vi "AutofocusOptions_old.vi"() -> ()   [LabVIEW 2019]
uses:
  <vilib>/Utility/file.llb/Read Delimited Spreadsheet (DBL).vi
panel:
  in  "DistSensorInTextFileMode":bool
  out "XYZ_NiterOrDistSenErr":string
  in  "AbortAutoFocus":bool
  in  "Tolerance":dbl=0.005 format="%#_13g"
  out "TimeTaken":dbl
  out "Z":string
  in  "SafeMaxZ":dbl=75.0 format="%#_13g"
  out "N_iterations":dbl[](array[numeric])
  in  "InitialStepSize":dbl=0.1
  out "HighVSPosition":picture
  in  "Z OutputFile":path=path "C:/Users/TTUHEP/Documents/LabVIEW/GantryPrograms/LogFiles/temp.txt"
  in  "PlotOutputFile":string="C:\\Users\\TTUHEP\\Documents\\LabVIEW\\GantryPrograms\\LogFiles\\plot.png"
  in  "Zoffset_textFile":dbl
  out "Image":T1(plugin-control)
  in  "InitialPositions":path=path "C:/Users/TTUHEP/Documents/LabVIEW/GantryPrograms/Configs/A1_BP_HeightMeasure.txt"
  out "error out":errorcluster
  out "BestZvalue":dbl
  in  "error in (no error)":errorcluster
  in  "Z":dbl=68.683
  in  "Y":dbl=1011.604463
  in  "X":dbl=288.7508563
  in  "ControlType":T2(ring)=enum."SinglePoint" caption="Operation Mode"
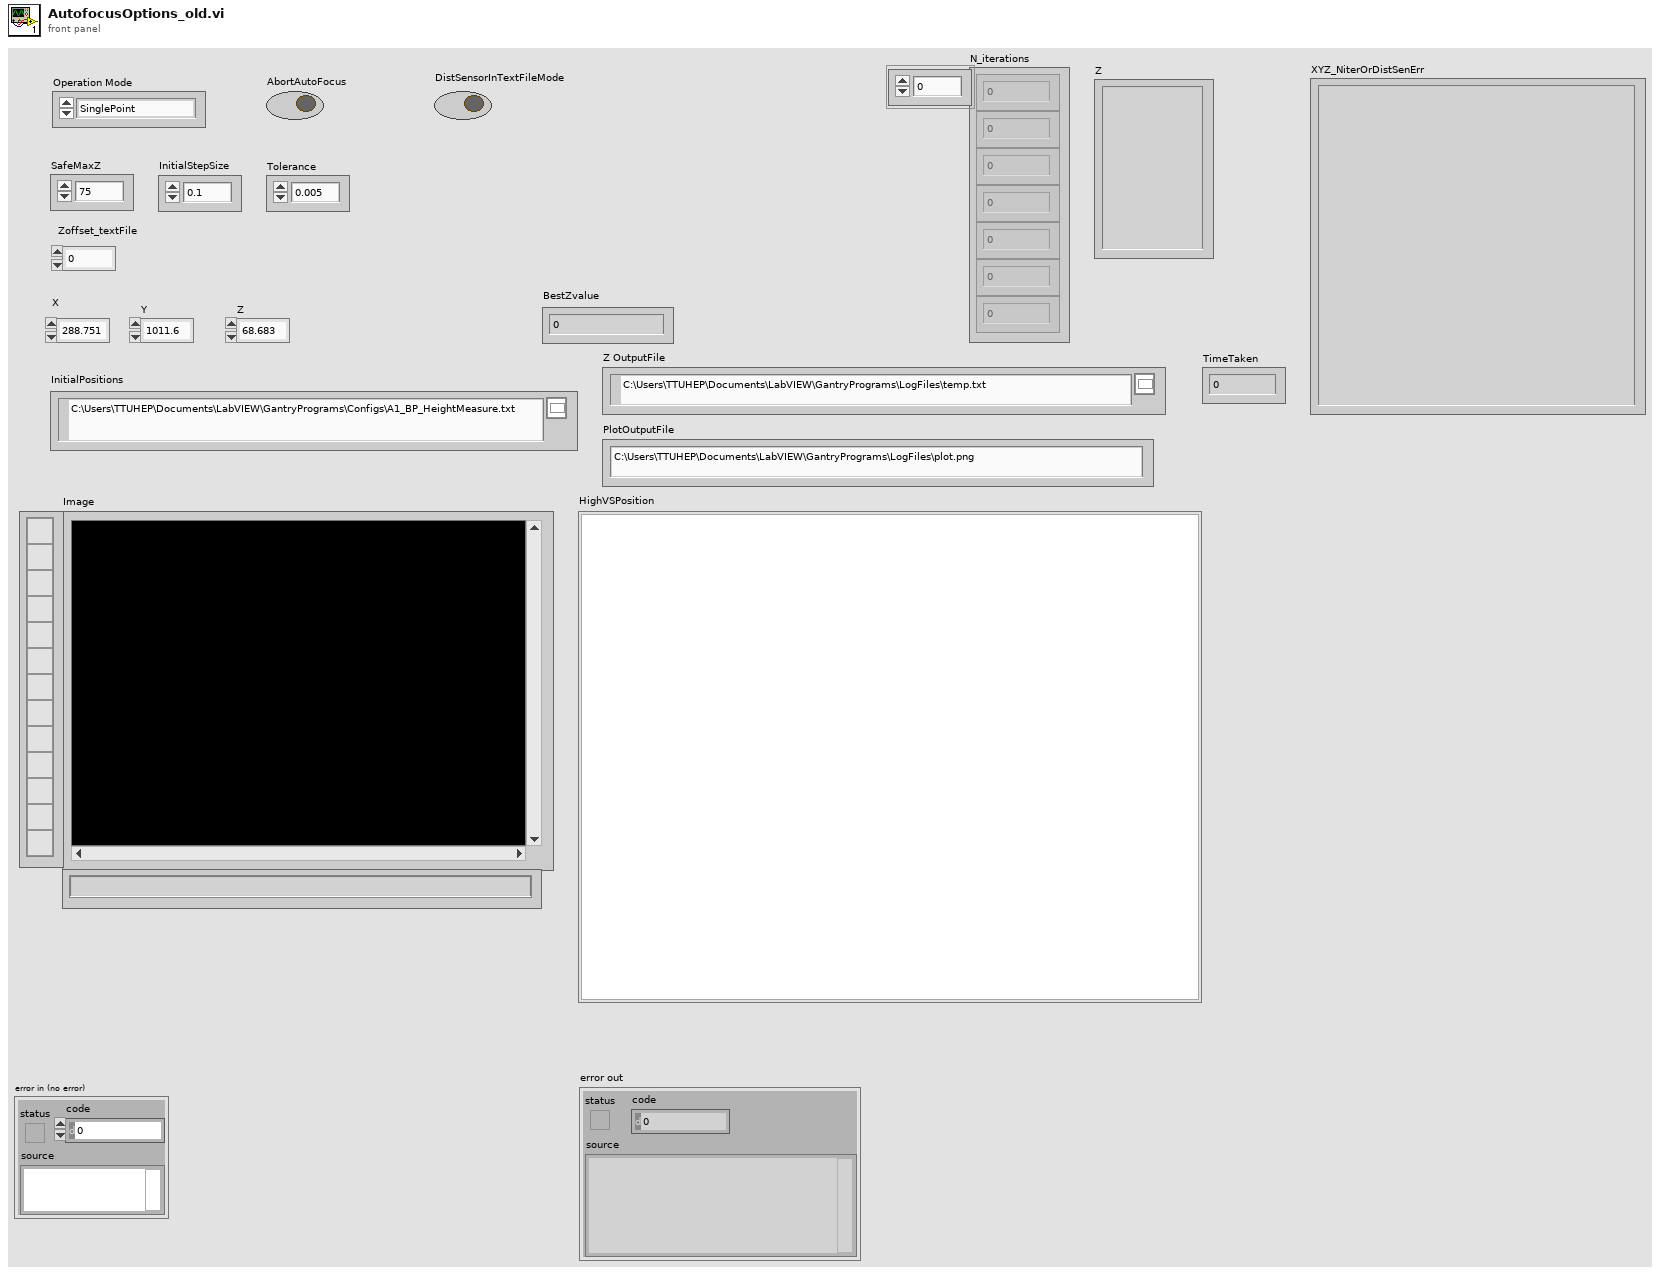
[diagram p1: front panel]
types:
  T1 = typedef "IMAQ Image.ctl" = refnum<image>
  T2 = enum16{"CurrentPosition", "SinglePoint", "TextFile"}
  T3 = enum16{"open", "replace", "create", "open or create", "replace or create", "replace or create with confirmation"}
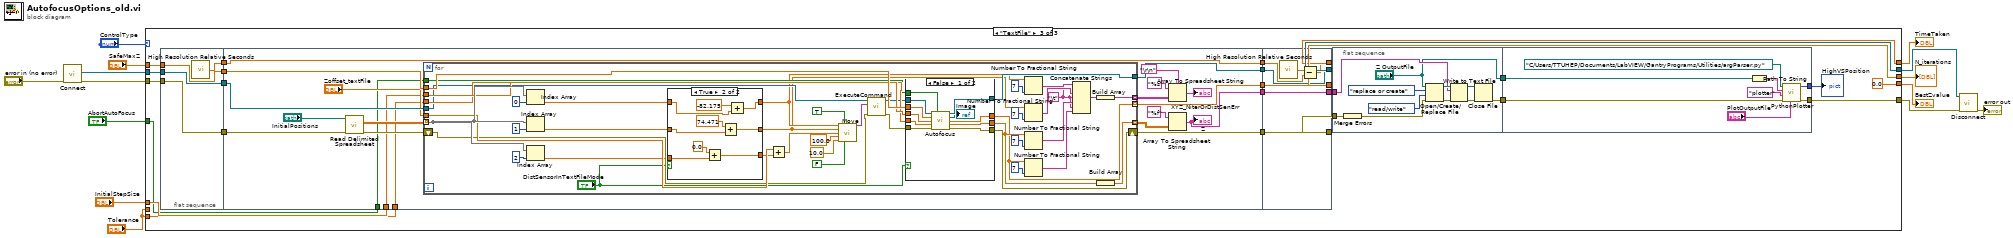
[diagram p0: block diagram]
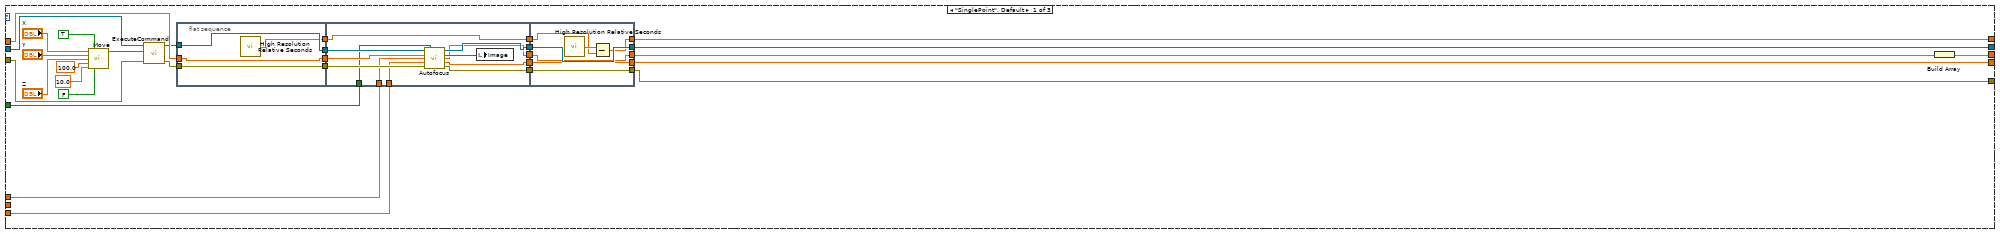
[diagram p2: hidden frame]
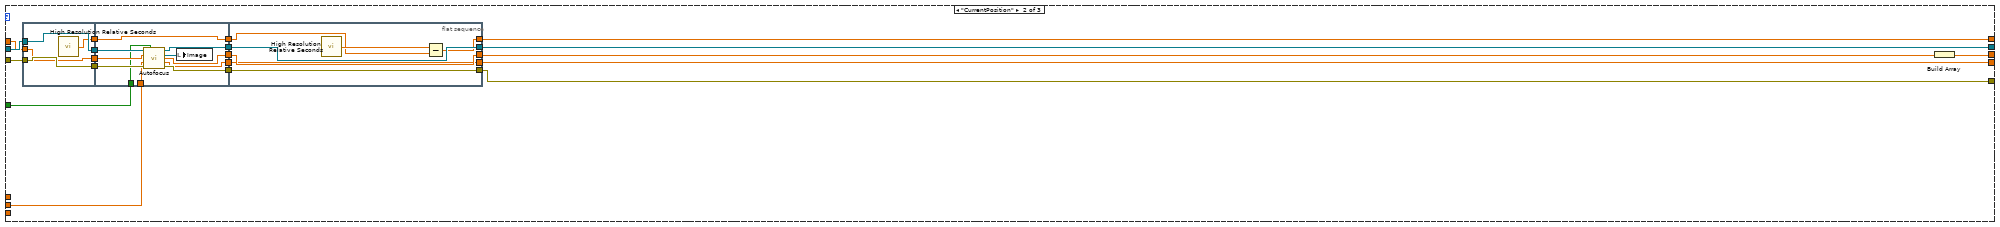
[diagram p3: hidden frame]
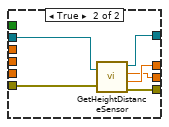
[diagram p4: hidden frame]
diagram:
  n1 = call "Connect.vi"("error in (no error)"="error in (no error)") -> ("error out"=w11:errorcluster, "controller"=w13:refnum<k24>)  [unwired: 9 in]
  n2 = case shown="\"TextFile\"" "ControlType" {
    tunnel: w11 -> [w19 w86 w130]
    tunnel: [w45 w82 w126] -> w10
    tunnel: w13 -> [w29 w87 w134]
    tunnel: [w44 w83 w133] -> w8
    tunnel: [w42 w84 w131] -> w7
    tunnel: "SafeMaxZ" -> [w41 w85 w129]
    tunnel: [w40 w81 0.0 ("BestZvalue")] -> w5
    tunnel: [w30 w71 w114] -> w4
    tunnel: "Tolerance" -> [_ w70 _]
    tunnel: "InitialStepSize" -> [w17 _ w113]
    tunnel: "Tolerance" -> [w16 _ w112]
    tunnel: "AbortAutoFocus" -> [w15 w69 w111]
    frame "SinglePoint", Default {
      n3 = call "Move.vi"("X"="X", "Absolute"=TRUE, "Y"="Y", "Z"="Z", "SpeedXY (mm/s)"=100.0, "SpeedZ (mm/s)"=10.0, "Move Z first"=FALSE) -> ("Position Gcode"=w20:string)  [unwired: 8 in]
      n4 = call "ExecuteCommand.vi"("error in (no error)"=w19, "Command Code"=w20, "controller in"=w29) -> ("error out"=w18:errorcluster, "controller out"=w28:refnum<k24>)  [unwired: 6 in, 1 out]
      n5 = flat-sequence {
        tunnel: w41 -> [w48]
        tunnel: w28 -> [w49]
        tunnel: [w46] -> w39
        tunnel: [w49] -> w38
        tunnel: [w48] -> w37
        tunnel: [w47] -> w31
        tunnel: w18 -> [w46]
        tunnel: w39 -> [w61]
        tunnel: w38 -> [w54]
        tunnel: w37 -> [w51]
        tunnel: [w60] -> w36
        tunnel: [w59] -> w35
        tunnel: [w57] -> w34
        tunnel: [w56] -> w33
        tunnel: [w55] -> w32
        tunnel: w31 -> [w55]
        tunnel: w17 -> [w53]
        tunnel: w16 -> [w52]
        tunnel: w15 -> [w50]
        tunnel: [w65] -> w40
        tunnel: [w66] -> w43
        tunnel: [w67] -> w44
        tunnel: [w68] -> w45
        tunnel: w36 -> [w68]
        tunnel: w35 -> [w67]
        tunnel: w34 -> [w66]
        tunnel: w33 -> [w65]
        tunnel: w32 -> [w63]
        tunnel: [w62] -> w30
        frame #0 {
          n6 = call <vilib>:"High Resolution Relative Seconds.vi"() -> ("relative seconds"=w47:dbl)
        }
        frame #1 {
          n7 = call "Autofocus.vi"("controller in"=w54, "AbortAutoFocus"=w50, "SafeMaxZ"=w51, "InitialStepSize"=w53, "Tolerance"=w52, "error in (no error)"=w61) -> ("controller out"=w59:refnum<k24>, "Image"=w58:T1, "N_iterations"=w57:dbl, "BestZvalue"=w56:dbl, "error out"=w60:errorcluster)  [unwired: 5 in]
          n8 = local write "Image"(w58) -> ()
        }
        frame #2 {
          n9 = call <vilib>:"High Resolution Relative Seconds.vi"() -> ("relative seconds"=w64:dbl)
          n10 = Subtract(x=w64, y=w63) -> (x-y=w62:dbl)
        }
      }
      n11 = Build Array(w43) -> (w42:dbl[])
    }
    frame "CurrentPosition" {
      n12 = flat-sequence {
        tunnel: w85 -> [w90]
        tunnel: w86 -> [w91]
        tunnel: w87 -> [w92]
        tunnel: [w92] -> w80
        tunnel: [w91] -> w79
        tunnel: [w90] -> w78
        tunnel: [w89] -> w73
        tunnel: w80 -> [w97]
        tunnel: w79 -> [w96]
        tunnel: w78 -> [w95]
        tunnel: [w102] -> w77
        tunnel: [w101] -> w76
        tunnel: [w100] -> w75
        tunnel: [w99] -> w74
        tunnel: w73 -> [w98]
        tunnel: [w98] -> w72
        tunnel: w70 -> [w94]
        tunnel: w69 -> [w93]
        tunnel: [w107] -> w81
        tunnel: [w108] -> w82
        tunnel: [w109] -> w83
        tunnel: [w110] -> w88
        tunnel: w77 -> [w110]
        tunnel: w76 -> [w109]
        tunnel: w75 -> [w108]
        tunnel: w74 -> [w107]
        tunnel: w72 -> [w105]
        tunnel: [w104] -> w71
        frame #0 {
          n13 = call <vilib>:"High Resolution Relative Seconds.vi"() -> ("relative seconds"=w89:dbl)
        }
        frame #1 {
          n14 = call "Autofocus.vi"("controller in"=w97, "AbortAutoFocus"=w93, "SafeMaxZ"=w95, "Tolerance"=w94, "error in (no error)"=w96) -> ("controller out"=w101:refnum<k24>, "Image"=w103:T1, "N_iterations"=w102:dbl, "BestZvalue"=w99:dbl, "error out"=w100:errorcluster)  [unwired: 6 in]
          n15 = local write "Image"(w103) -> ()
        }
        frame #2 {
          n16 = call <vilib>:"High Resolution Relative Seconds.vi"() -> ("relative seconds"=w106:dbl)
          n17 = Subtract(x=w106, y=w105) -> (x-y=w104:dbl)
        }
      }
      n18 = Build Array(w88) -> (w84:dbl[])
    }
    frame "TextFile" {
      n19 = flat-sequence {
        tunnel: w129 -> [w137]
        tunnel: w130 -> [w138]
        tunnel: w134 -> [w139]
        tunnel: [w139] -> w123
        tunnel: [w138] -> w122
        tunnel: [w137] -> w121
        tunnel: [w136] -> w116
        tunnel: w123 -> [w158]
        tunnel: w122 -> [w154]
        tunnel: w121 -> [w152]
        tunnel: [w140] -> w120
        tunnel: [w157] -> w119
        tunnel: [w141] -> w118
        tunnel: [w155] -> w117
        tunnel: w116 -> [w149]
        tunnel: [w149] -> w115
        tunnel: w113 -> [w148]
        tunnel: w112 -> [w147]
        tunnel: w111 -> [w146]
        tunnel: [w235] -> w131
        tunnel: [w236] -> w132
        tunnel: [w237] -> w133
        tunnel: [w238] -> w135
        tunnel: w120 -> [w238]
        tunnel: w119 -> [w237]
        tunnel: w118 -> [w236]
        tunnel: w117 -> [w235]
        tunnel: w115 -> [w233]
        tunnel: [w232] -> w114
        frame #0 {
          n20 = call <vilib>:"High Resolution Relative Seconds.vi"() -> ("relative seconds"=w136:dbl)
        }
        frame #1 {
          n21 = call-poly <vilib>:"Read Delimited Spreadsheet.vi"("file path (dialog if empty)"="InitialPositions", "error in (no error)"=w154) -> ("all rows"=w160:dbl[][], "error out"=w153:errorcluster)  [unwired: 8 in, 4 out]
          n22 = for {
            tunnel: w160 -> [w199] mode=indexing
            tunnel: [w198] -> w150 mode=indexing
            tunnel: w158 -> [w184]
            tunnel: [w197] -> w157
            tunnel: [w163] -> w155 mode=indexing
            tunnel: w152 -> [w187]
            tunnel: "Zoffset_textFile" -> [w196]
            tunnel: w148 -> [w186]
            tunnel: w147 -> [w185]
            tunnel: w146 -> [w182]
            tunnel: [w173] -> w145 mode=indexing
            shift-right: [w172] -> w140
            shift-left: w153 -> [w189]
            w164 = "\t"
            n23 = Index Array(array=w199, index=0) -> (element=w170:dbl)
            n24 = Index Array(array=w199, index=1) -> (element=w168:dbl)
            n25 = Index Array(array=w199, index=2) -> (element=w167:dbl)
            n26 = case shown="True" "DistSensorInTextFileMode" {
              tunnel: [w222 w230] -> w171
              tunnel: w170 -> [w222 w229]
              tunnel: [w221 w228] -> w169
              tunnel: w168 -> [w221 w226]
              tunnel: w167 -> [w220 w225]
              tunnel: [w220 w223] -> w166
              frame False {
              }
              frame True {
                n27 = Add(x=0.0, y=w225) -> (x+y=w223:dbl)
                n28 = Add(x=74.471, y=w226) -> (x+y=w228:dbl)
                n29 = Add(x=-82.175, y=w229) -> (x+y=w230:dbl)
              }
            }
            n30 = Add(x=w196, y=w166) -> (x+y=w195:dbl)
            n31 = call "Move.vi"("X"=w171, "Absolute"=TRUE, "Y"=w169, "Z"=w195, "SpeedXY (mm/s)"=100.0, "SpeedZ (mm/s)"=10.0, "Move Z first"=FALSE) -> ("Position Gcode"=w190:string)  [unwired: 8 in]
            n32 = call "ExecuteCommand.vi"("error in (no error)"=w189, "Command Code"=w190, "controller in"=w184) -> ("error out"=w188:errorcluster, "controller out"=w183:refnum<k24>)  [unwired: 6 in, 1 out]
            n33 = case shown="False" "DistSensorInTextFileMode" {
              tunnel: [w213 w217] -> w197
              tunnel: [w212 w215] -> w163
              tunnel: w188 -> [w210 w218]
              tunnel: w187 -> [w209 _]
              tunnel: w186 -> [w208 _]
              tunnel: w185 -> [w207 _]
              tunnel: w183 -> [w206 w219]
              tunnel: w182 -> [w205 _]
              tunnel: [w204 w214] -> w179
              tunnel: [w203 w216] -> w172
              frame False {
                n34 = call "Autofocus.vi"("controller in"=w206, "AbortAutoFocus"=w205, "SafeMaxZ"=w209, "InitialStepSize"=w208, "Tolerance"=w207, "error in (no error)"=w210) -> ("controller out"=w213:refnum<k24>, "Image"=→"Image":T1, "N_iterations"=w212:dbl, "BestZvalue"=w204:dbl, "error out"=w203:errorcluster)  [unwired: 5 in]
              }
              frame True {
                n35 = call "GetHeightDistanceSensor.vi"("controller in"=w219, "error in (no error)"=w218) -> ("controller out"=w217:refnum<k24>, "MeanHeight(mm)"=w214:dbl, "SDofHeight(mm)"=w215:dbl, "error out"=w216:errorcluster)
              }
            }
            n36 = Number To Fractional String(number=w171, precision (6)=i16 7) -> (F-format string=w177:string)  [unwired: 2 in]
            n37 = Number To Fractional String(number=w169, precision (6)=i16 7) -> (F-format string=w176:string)  [unwired: 2 in]
            n38 = Number To Fractional String(number=w179, precision (6)=i16 7) -> (F-format string=w175:string)  [unwired: 2 in]
            n39 = Number To Fractional String(number=w163, precision (6)=i16 7) -> (F-format string=w161:string)  [unwired: 2 in]
            n40 = Concatenate Strings(w177, w164, w176, w164, w175, w164, w161) -> (w174:string)
            n41 = Build Array(w174) -> (w173:string[])
            n42 = Build Array(w179) -> (w198:dbl[])
          }
          n43 = Array To Spreadsheet String(array=w150, 3:"%f" ("format string")) -> (spreadsheet string=w141:string)  [unwired: 1 in]
          "Z" <- w141
          n44 = Array To Spreadsheet String(delimiter (Tab)="\r\n", array=w145, 3:"%s" ("format string")) -> (spreadsheet string=→"XYZ_NiterOrDistSenErr":string)
        }
        frame #2 {
          n45 = call <vilib>:"High Resolution Relative Seconds.vi"() -> ("relative seconds"=w234:dbl)
          n46 = Subtract(x=w234, y=w233) -> (x-y=w232:dbl)
        }
      }
      n47 = flat-sequence {
        tunnel: w135 -> [w249]
        tunnel: w132 -> [w242]
        tunnel: [w240] -> w127
        tunnel: ["Z OutputFile"] -> w124
        tunnel: w127 -> [w257]
        tunnel: [w256] -> w126
        tunnel: [w255] -> w125
        tunnel: w124 -> [w251]
        frame #0 {
          n48 = Merge Errors(w249) -> (w241:errorcluster)
          n49 = Open/Create/Replace File(file path (use dialog)="Z OutputFile", error in=w241, operation (0:open)=T3."replace or create", access (0:read/write)=enum16{"read/write", "read-only", "write-only"}."read/write") -> (refnum out=w245:refnum<file>, error out=w246:errorcluster)  [unwired: 2 in, 1 out]
          n50 = Write to Text File(file (use dialog)=w245, text=w242, error in=w246) -> (refnum out=w248:refnum<file>, error out=w247:errorcluster)  [unwired: 1 in, 1 out]
          n51 = Close File(refnum=w248, error in=w247) -> (error out=w240:errorcluster)  [unwired: 1 out]
        }
        frame #1 {
          n52 = Path To String(path=w251) -> (string=w252:string)
          n53 = call "PythonPlotter.vi"("Output File"="PlotOutputFile", "error in (no error)"=w257, "Function Name"="plotter", "Input File"=w252, "Python Path"=path "C:/Users/TTUHEP/Documents/LabVIEW/GantryPrograms/Utilities/argParser.py") -> ("error out"=w256:errorcluster, "HighVSPosition"=w255:picture)  [unwired: 4 in]
        }
      }
      "HighVSPosition" <- w125
    }
  }
  "N_iterations" <- w7
  "BestZvalue" <- w5
  "TimeTaken" <- w4
  n54 = call "Disconnect.vi"("error in (no error)"=w10, "controller"=w8) -> ("error out"=→"error out":errorcluster)  [unwired: 9 in]
